vi "GetAllIsometriesOf2DArray.vi"(8 "error in (no error)":errorcluster, 11 "Array In":i8[][](array[numeric])) -> (0 "error out":errorcluster, 3 "All Isometrioes Out":i8[][][](array[numeric]))   [LabVIEW 2020]
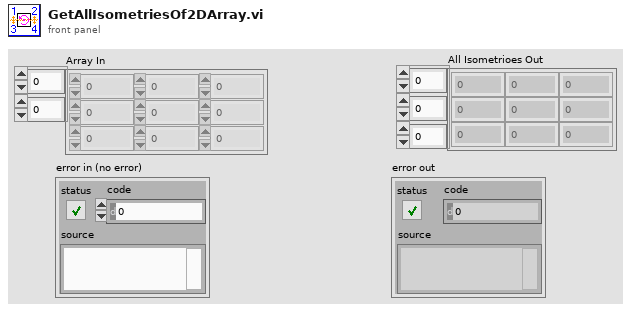
[diagram p1: front panel]
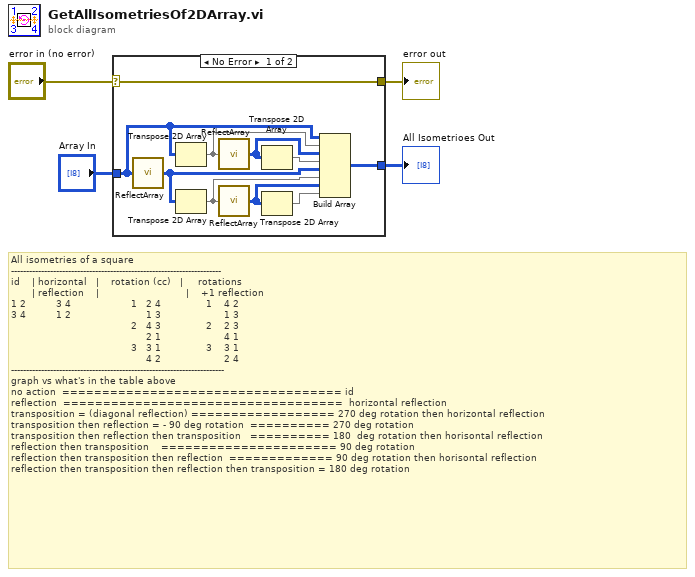
[diagram p0: block diagram]
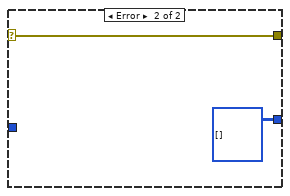
[diagram p2: hidden frame]
diagram:
  # "All isometries of a square\n----------------------------------------------------------------------\nid    | horizontal   |    rotation (cc)   |     rotations\n       | reflection    |                             |    +1 reflection\n1 2          3 4                    1   2 4               1    4 2\n3 4          1 2                         1 3                     1 3\n                                        2   4 3               2    2 3\n                                             2 1                     4 1\n                                        3   3 1               3    3 1 \n                                             4 2                     2 4\n-----------------------------------------------------------------------\ngraph vs what's in the table above\nno action  =================================== id \nreflection  ===================================  horizontal reflection\ntransposition = (diagonal reflection) ================== 270 deg rotation then horizontal reflection\ntransposition then reflection = - 90 deg rotation  ========== 270 deg rotation\ntransposition then reflection then transposition   ========== 180  deg rotation then horisontal reflection \nreflection then transposition    ====================== 90 deg rotation\nreflection then transposition then reflection  ============= 90 deg rotation then horisontal reflection\nreflection then transposition then reflection then transposition = 180 deg rotation"
  n1 = case shown="No Error" "error in (no error)" {
    selector: "error in (no error)" -> [w14 w16]
    tunnel: "Array In" -> [w13 _]
    tunnel: [w12 i8[][][] []] -> w3
    tunnel: [w14 w16] -> w1
    frame No Error {
      n2 = call "ReflectArray.vi"("Array in"=w13) -> ("Array out"=w8:i8[][])  [unwired: 4 in]
      n3 = Transpose 2D Array(2D array=w13) -> (transposed array=w11:i8[][])
      n4 = Transpose 2D Array(2D array=w8) -> (transposed array=w7:i8[][])
      n5 = call "ReflectArray.vi"("Array in"=w11) -> ("Array out"=w10:i8[][])  [unwired: 4 in]
      n6 = call "ReflectArray.vi"("Array in"=w7) -> ("Array out"=w6:i8[][])  [unwired: 4 in]
      n7 = Transpose 2D Array(2D array=w10) -> (transposed array=w9:i8[][])
      n8 = Transpose 2D Array(2D array=w6) -> (transposed array=w5:i8[][])
      n9 = Build Array(w13, w11, w10, w9, w8, w7, w6, w5) -> (w12:i8[][][])
    }
    frame Error {
    }
  }
  "All Isometrioes Out" <- w3
  "error out" <- w1
